vi "MVE Custom TD.vi"() -> (0 "errorMsg":string, 1 "error?":bool, 2 "typeDescriptor":u8[](array[numeric]), 3 "Cancelled":bool)   [LabVIEW 2016]
uses:
  <vilib>/Utility/error.llb/DialogType.ctl
  Instance           1 21Saved   MVE Custom TD .vi
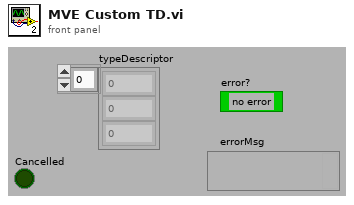
[diagram p1: front panel]
types:
  T1 = typedef "DialogType.ctl" = u16
  T2 = typedef "NI_Variable.lvlib/Type Descriptor.ctl" = cluster{"Variant":variant}
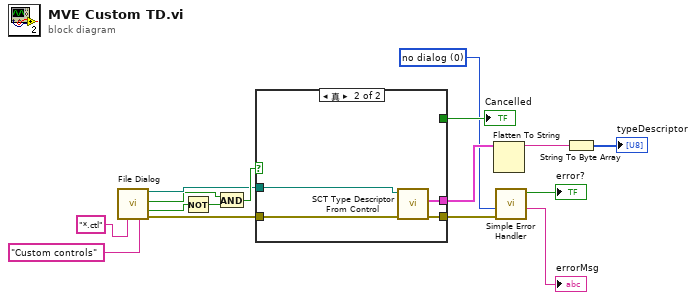
[diagram p0: block diagram]
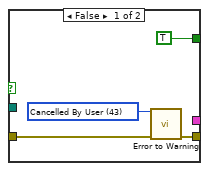
[diagram p2: hidden frame]
diagram:
  w3 = T1 0 items=["no dialog", "OK message", "continue or stop message", "OK message + warnings", "continue/stop + warnings"] ("type of dialog (OK msg:1)")
  n1 = call "File Dialog"("pattern (all files)"="*.ctl", "pattern label"="Custom controls") -> ("selected path"=w8:path, "exists"=w4:bool, "cancelled"=w5:bool, "error out"=w9:errorcluster)  [unwired: 10 in]
  n2 = Not(x=w5) -> (.not. x?=w15:bool)
  n3 = And(x=w4, y=w15) -> (x .and. y?=w16:bool)
  n4 = case shown="真" w16 {
    tunnel: w8 -> [_ w24]
    tunnel: w9 -> [w19 w23]
    tunnel: [_ w22] -> w11
    tunnel: [w18 w21] -> w14
    tunnel: [TRUE _] -> w13
    frame False {
      w17 = 43 items=["No Error", "Argument Error", "Memory Full", "Out of Zone", "End of File", "File Already Open", "Generic File IO Error", "File Not Found", "File Permission Error", "Disk Full", "Duplicate Path", "Too Many Files Open", "Not Enabled", "Resource File Not Found", "Cannot Add Resource", "Resource Not Found", "Image Not Found", "Image Memory Error", "Pen Does Not Exist", "Config Bad Type", "Config Token Not Found", "Config Parse Error", "Config Memory Error", "Bad External Code Format", "Bad External Code Offset", "External Code Not Present", "Null Window", "Destroy Window Mixup", "Null Menu", "Print Aborted", "Bad Print Record", "Print Driver Error", "Windows Error During Print", "Memory Error During Print", "Print Dialog Error", "Generic Print Error", "Invalid Device Refnum", "Device Not Found", "Device Parameter Error", "Device Unit Error", "Can't Open Device", "Device Call Aborted", "Generic Error", "Cancelled By User", "Object ID Too Low", "Object ID Too High", "Object Not In Heap", "Unknown Heap", "Bad DefProc ID", "DefProc Not In Table", "Message Out Of Range", "Null Method", "Unknown Message", "Manager Call Not Supported", "Bad address", "Connection In progress", "Connection timed out", "Connection is already in progress", "Network attribute not supported", "Network error", "Address in use", "System out of memory", "Connection aborted", "Connection refused", "Connection is not connected", "Connection is already connected", "Connection closed", "Initialize error (interapplication manager)", "Bad occurrence", "Wait on unbound occurrence handler", "Occurrence queue overflow", "Bad path", "Semaphore not signaled", "Unrecognized type (interapplication manager)"] ("1st Error to Convert")
      n5 = call <vilib>:"Error to Warning.vi"("1st Error to Convert"=w17, "error in"=w19) -> ("warning out"=w18:errorcluster)  [unwired: 13 in]
    }
    frame True {
      n6 = call <resource>:"SCT Type Descriptor From Control.vi"("error in (no error)"=w23, "custom type path"=w24) -> ("error out"=w21:errorcluster, "type descriptor"=w22:T2)  [unwired: 7 in, 1 out]
    }
  }
  "Cancelled" <- w13
  n7 = Flatten To String(anything=w11) -> (data string=w10:string)  [unwired: 3 in, 2 out]
  n8 = call <vilib>:"Simple Error Handler.vi"("type of dialog (OK msg:1)"=w3, "error in (no error)"=w14) -> ("error?"=→"error?":bool, "source out"=→"errorMsg":string)  [unwired: 3 in, 3 out]
  n9 = String To Byte Array(string=w10) -> (unsigned byte array=→"typeDescriptor":u8[])
